vi "embeddedREPL.vi"() -> ()   [LabVIEW 2019]
uses:
  <userlib>/MicroPython/VIs/uPythonX/PythonData.ctl
  <userlib>/MicroPython/VIs/uPythonX/uPythonX.xctl
panel:
  in  "Code":string
  in  "Control Name":string="Robot REPL"
  in  "Data In":T1={"Port"="", "All Code"="Hi"}
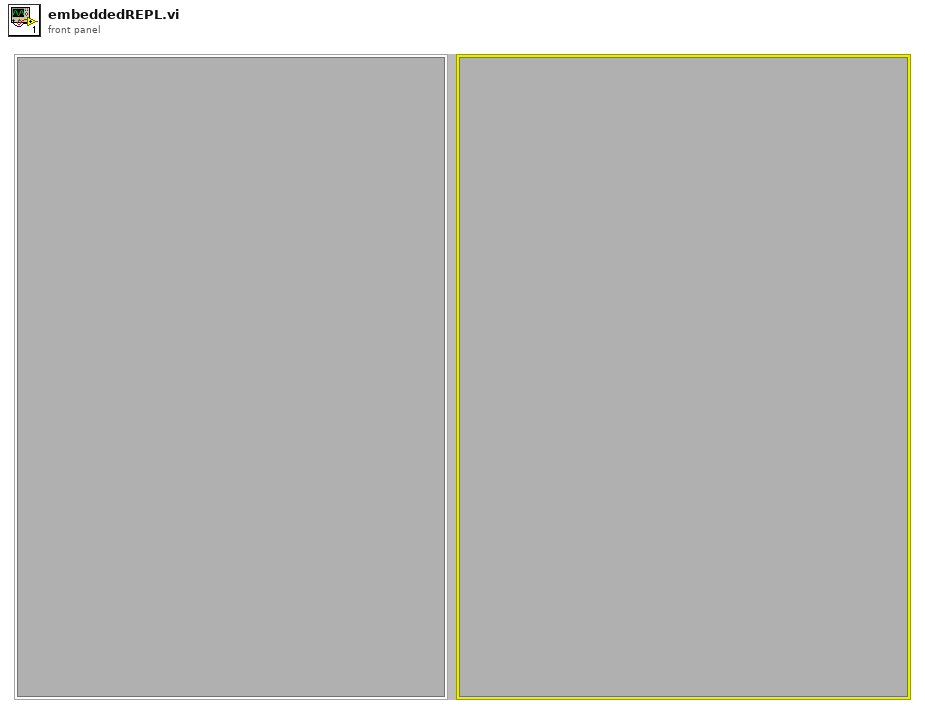
[diagram p1: front panel]
types:
  T1 = typedef "uPythonX.xctl/PythonData.ctl" = cluster{"Port":refnum<visa-resource-name>, "All Code":string}
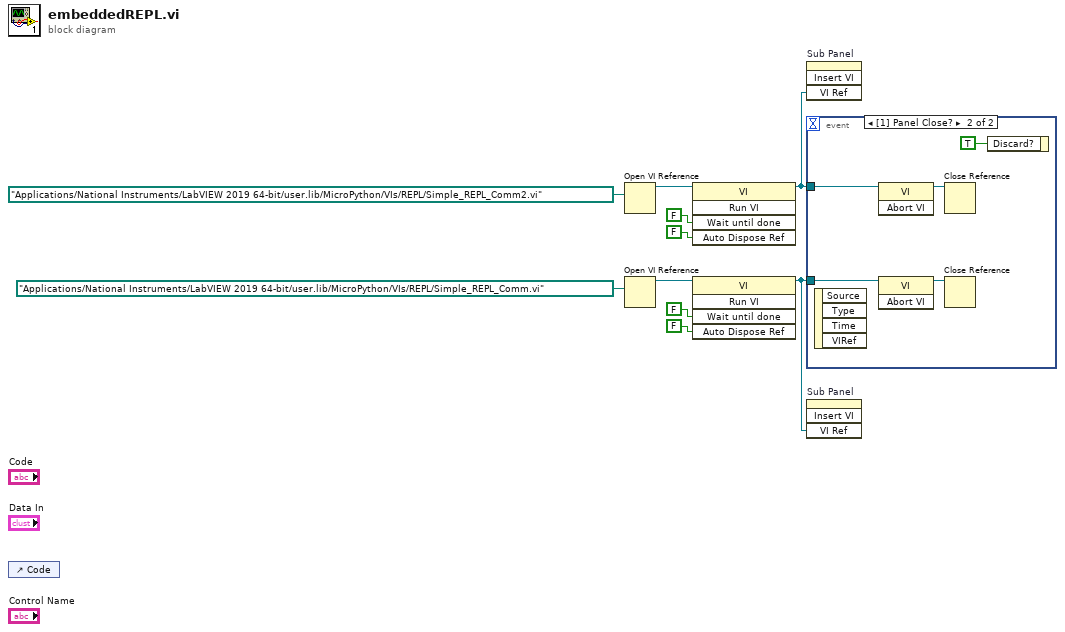
[diagram p0: block diagram]
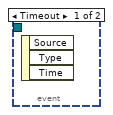
[diagram p2: hidden frame]
diagram:
  n1 = control-ref of="Code"() -> ()  [unwired: 1 out]
  n2 = Open VI Reference(vi path=path "/Applications/National Instruments/LabVIEW 2019 64-bit/user.lib/MicroPython/VIs/REPL/Simple_REPL_Comm2.vi" ("Name")) -> (vi reference=w2:refnum<vi>)  [unwired: 5 in, 1 out]
  n3 = Open VI Reference(vi path=path "/Applications/National Instruments/LabVIEW 2019 64-bit/user.lib/MicroPython/VIs/REPL/Simple_REPL_Comm.vi" ("Name")) -> (vi reference=w10:refnum<vi>)  [unwired: 5 in, 1 out]
  n4 = invoke class="VI" method="Run VI"(reference=w2, "Wait until done"=FALSE ("Wait Until Done"), "Auto Dispose Ref"=FALSE ("Auto Dispose Reference")) -> (reference out=w1:refnum<vi>)  [unwired: 2 in, 4 out]
  n5 = invoke class="VI" method="Run VI"(reference=w10, "Wait until done"=FALSE ("Wait Until Done"), "Auto Dispose Ref"=FALSE ("Auto Dispose Reference")) -> (reference out=w8:refnum<vi>)  [unwired: 2 in, 4 out]
  n6 = invoke on="Sub Panel" class="SubPnl" method="Insert VI"("VI Ref"=w1) -> ()  [unwired: 3 in, 4 out]
  n7 = event shown="[1] Panel Close?" {
    selector: _ -> [_ _]
    dyn-events: _ -> [_ _]
    timeout: _ -> [_ _]
    tunnel: w8 -> [_ w14]
    tunnel: w1 -> [_ w12]
    event Timeout {
      n8 = event-data() -> ()  [unwired: 1 in, 3 out]
    }
    event Panel Close? {
      n9 = event-data() -> ()  [unwired: 1 in, 4 out]
      n10 = invoke class="VI" method="Abort VI"(reference=w12) -> (reference out=w11:refnum<vi>)  [unwired: 2 in, 2 out]
      n11 = invoke class="VI" method="Abort VI"(reference=w14) -> (reference out=w13:refnum<vi>)  [unwired: 2 in, 2 out]
      n12 = Close Reference(reference=w11) -> ()  [unwired: 1 in, 1 out]
      n13 = Close Reference(reference=w13) -> ()  [unwired: 1 in, 1 out]
      n14 = event-data("Discard?"=TRUE) -> ()  [unwired: 1 in, 1 out]
    }
  }
  n15 = invoke on="Sub Panel" class="SubPnl" method="Insert VI"("VI Ref"=w8) -> ()  [unwired: 3 in, 4 out]
